vi "Lift.vi"(9 "Up Button":bool, 10 "Down Button":bool) -> (2 "Brake State":T1=enum."Forward", 3 "Lift Motor":dbl)   [LabVIEW 2014]
uses:
  <vilib>/Rock Robotics/WPI/Solenoid/WPI_SolenoidValue.ctl
  Robot Global Data.vi
  <vilib>/Rock Robotics/WPI/Solenoid/WPI_SolenoidGetEnum.vi
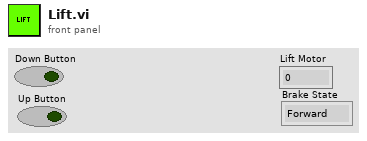
[diagram p1: front panel]
types:
  T1 = typedef "WPI_SolenoidValue.ctl" = enum16{"Off", "On", "Forward", "Reverse"}
  T2 = typedef "WPI_SolenoidDevRef.ctl" = cluster{"DevStatus":errorcluster, "Pneumatics Control Module":u8, "Forward Solenoid Channel":T3, "Reverse Solenoid Channel":T3}
  T3 = typedef "WPI_SolenoidChannel.ctl" = enum8{"Solenoid 0", "Solenoid 1", "Solenoid 2", "Solenoid 3", "Solenoid 4", "Solenoid 5", "Solenoid 6", "Solenoid 7", "Invalid"}
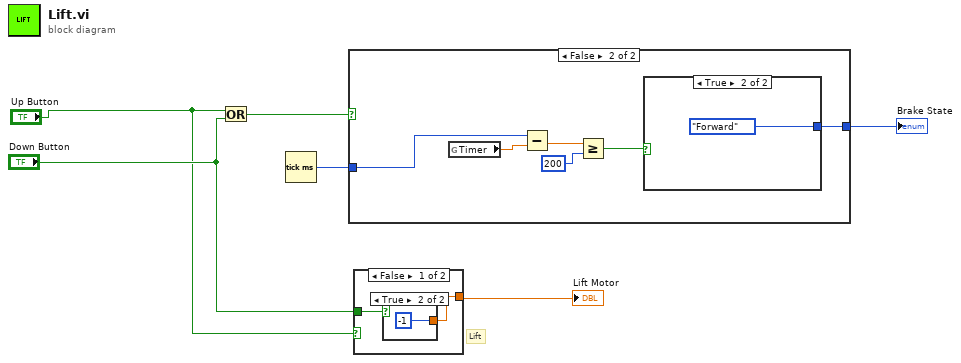
[diagram p0: block diagram]
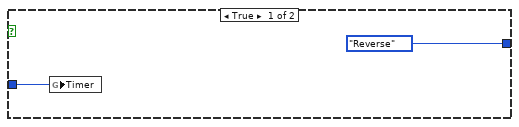
[diagram p2: hidden frame]
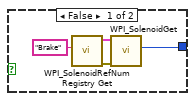
[diagram p3: hidden frame]
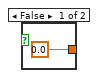
[diagram p4: hidden frame]
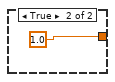
[diagram p5: hidden frame]
diagram:
  # "Lift"
  n1 = Or(x="Up Button", y="Down Button") -> (x .or. y?=w3:bool)
  n2 = Tick Count (ms)() -> (millisecond timer value=w2:u32)
  n3 = case shown="False" w3 {
    tunnel: w2 -> [w8 w13]
    tunnel: [WPI_SolenoidValue."Reverse" ("Value") w9] -> w1
    frame True {
      n4 = global write "Robot Global Data.vi" "Timer"(w8) -> ()
    }
    frame False {
      n5 = global read "Robot Global Data.vi" "Timer"() -> (w14:dbl)
      n6 = Subtract(x=w13, y=w14) -> (x-y=w11:dbl)
      n7 = Greater Or Equal?(x=w11, y=u32 200) -> (x >= y?=w10:bool)
      n8 = case shown="True" w10 {
        tunnel: [w15 WPI_SolenoidValue."Forward" ("Value")] -> w9
        frame False {
          n9 = call <vilib>:"WPI_SolenoidRefNum Registry Get.vi"("refnum name"="Brake") -> ("error out"=w18:errorcluster, "SolenoidDevRef"=w17:T2)  [unwired: 9 in]
          n10 = call-poly <vilib>:"WPI_SolenoidGet.vi"("error in (no error)"=w18, "SolenoidDevRef"=w17) -> ("Value"=w15:T1)  [unwired: 7 in, 2 out]
        }
        frame True {
        }
      }
    }
  }
  "Brake State" <- w1
  n11 = case shown="False" "Up Button" {
    tunnel: [w21 1.0 ("f")] -> w6
    tunnel: "Down Button" -> [w20 _]
    frame False {
      n12 = case shown="True" w20 {
        tunnel: [0.0 -1] -> w21
        frame False {
        }
        frame True {
        }
      }
    }
    frame True {
    }
  }
  "Lift Motor" <- w6
